vi "VSI Flash Init.vi"(9 "pFlashInitConfig":T1, 10 "DevIndex":i32, 11 "DevType":i32) -> (1 "pFlashInitConfig out":T1, 3 "function return":i32)   [LabVIEW 2010, in "ControlSPI.lvlib"]
doc: "int WINAPI VSI_FlashInit(int DevType,int DevIndex, PVSI_FLASH_INIT_CONFIG pFlashInitConfig);"
uses:
  ControlSPI.lvlib
  ControlSPI/Ginkgo_Driver.dll
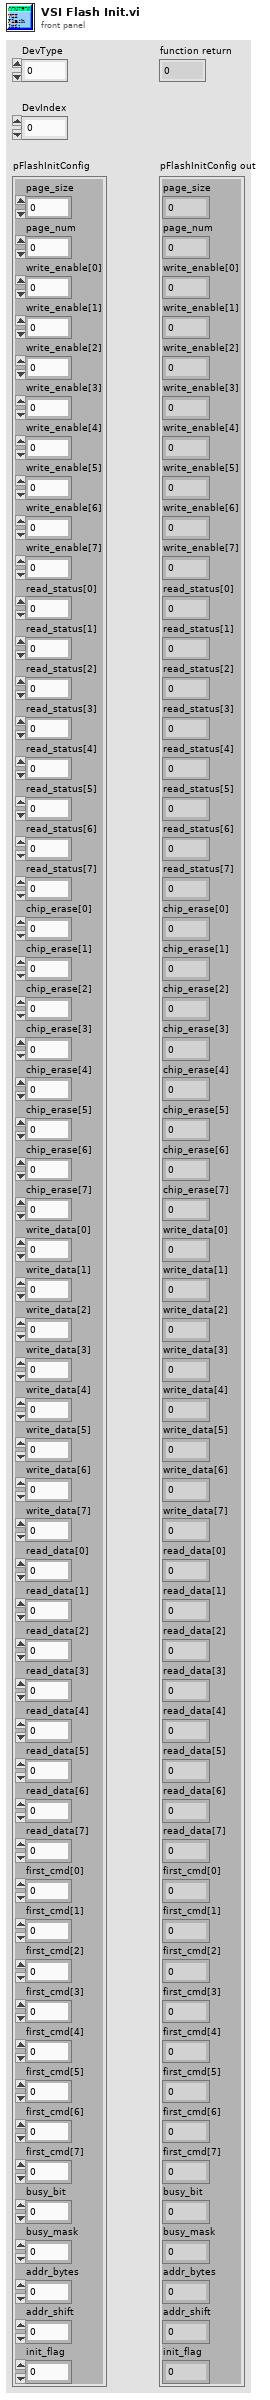
[diagram p1: front panel]
types:
  T1 = cluster{"page_size":u32, "page_num":u32, "write_enable[0]":u8, "write_enable[1]":u8, "write_enable[2]":u8, "write_enable[3]":u8, "write_enable[4]":u8, "write_enable[5]":u8, "write_enable[6]":u8, "write_enable[7]":u8, "read_status[0]":u8, "read_status[1]":u8, "read_status[2]":u8, "read_status[3]":u8, "read_status[4]":u8, "read_status[5]":u8, "read_status[6]":u8, "read_status[7]":u8, "chip_erase[0]":u8, "chip_erase[1]":u8, "chip_erase[2]":u8, "chip_erase[3]":u8, "chip_erase[4]":u8, "chip_erase[5]":u8, "chip_erase[6]":u8, "chip_erase[7]":u8, "write_data[0]":u8, "write_data[1]":u8, "write_data[2]":u8, "write_data[3]":u8, "write_data[4]":u8, "write_data[5]":u8, "write_data[6]":u8, "write_data[7]":u8, "read_data[0]":u8, "read_data[1]":u8, "read_data[2]":u8, "read_data[3]":u8, "read_data[4]":u8, "read_data[5]":u8, "read_data[6]":u8, "read_data[7]":u8, "first_cmd[0]":u8, "first_cmd[1]":u8, "first_cmd[2]":u8, "first_cmd[3]":u8, "first_cmd[4]":u8, "first_cmd[5]":u8, "first_cmd[6]":u8, "first_cmd[7]":u8, "busy_bit":u8, "busy_mask":u8, "addr_bytes":u8, "addr_shift":u8, "init_flag":u8}
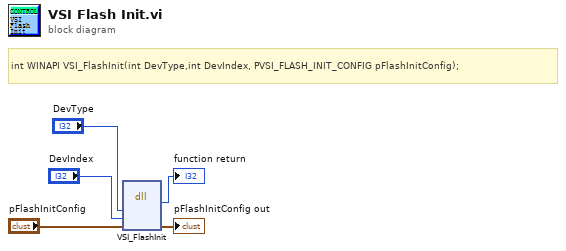
[diagram p0: block diagram]
diagram:
  # "int WINAPI VSI_FlashInit(int DevType,int DevIndex, PVSI_FLASH_INIT_CONFIG pFlashInitConfig);"
  n1 = dll-call lib="E:/Project/vt_ginkgo/truck/Ginkgo Driver/vs2010/Ginkgo_USB-I2C&SPI&CAN_API_v2.0.3.3/lib/labview_32bit/ControlSPI/Ginkgo_Driver.*" fn="VSI_FlashInit"("DevType"="DevType", "DevIndex"="DevIndex", "pFlashInitConfig"="pFlashInitConfig") -> (→"function return":i32, "pFlashInitConfig"=→"pFlashInitConfig out":T1)  [unwired: 5 in, 2 out]
